vi "Get System Resources.vi"(8 "error in":errorcluster, 11 "Session in":refnum<k21>="localhost") -> (0 "error out":errorcluster, 1 "System Summary":T1, 2 "System Resources":T2, 3 "Session out":refnum<k21>="localhost")   [LabVIEW 2016]
uses:
  Controls/SystemResources.ctl
  Controls/CPULoad.ctl
  <resource>/objmgr/nisysapi.rc
  RT Management.lvclass
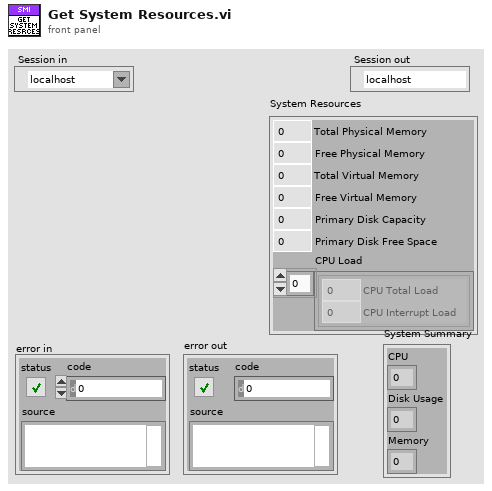
[diagram p1: front panel]
types:
  T1 = cluster{"CPU":dbl, "Disk Usage":dbl, "Memory":dbl}
  T2 = typedef "RT Management.lvlib/RT Management.lvclass/SystemResources.ctl" = cluster{"Total Physical Memory":dbl, "Free Physical Memory":dbl, "Total Virtual Memory":dbl, "Free Virtual Memory":dbl, "Primary Disk Capacity":dbl, "Primary Disk Free Space":dbl, "CPU Load":T3[]}
  T3 = typedef "RT Management.lvlib/RT Management.lvclass/CPULoad.ctl" = cluster{"CPU Total Load":dbl, "CPU Interrupt Load":dbl}
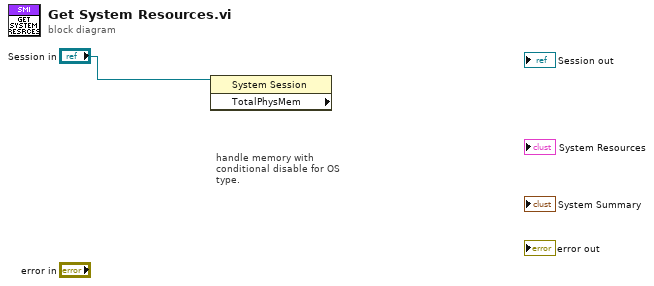
[diagram p0: block diagram]
diagram:
  # "handle memory with\nconditional disable for OS\ntype."
  n1 = property class="System Session" props=["TotalPhysMem"](reference="Session in") -> ()  [unwired: 1 in, 3 out]
